vi "Roller Loop.vi"(11 "Reset Pots?":bool) -> (3 "first run complete?":bool)   [LabVIEW 2014]
uses:
  Common Code/Roller Indicators.ctl
  Common Code/Roller Mode Enum.ctl
  Common Code/Auto Roller Commands.ctl
  Common Code/Inner Roller States.ctl
  Sensors/Pot Data.ctl
  Untip Can States.ctl
  Roller Modes.ctl
  Really Real Manual Align.ctl
  Common Code/Change Detect Int.vi
  Robot Global Data.vi
  <vilib>/Rock Robotics/WPI/Solenoid/Deprecated/WPI_SolenoidSetBool.vi
  <vilib>/Rock Robotics/WPI/DriverStation/WPI_DriverStationRobotMode2.ctl
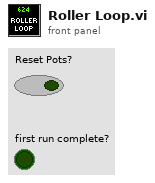
[diagram p1: front panel]
types:
  T1 = typedef "Roller Modes.ctl" = cluster{"Auto Roller Command":T2, "Roller Mode":T3, "Override Speed":dbl}
  T2 = typedef "Auto Roller Commands.ctl" = enum16{"Drag Tote", "Grab Tote", "Idle", "Eject Tote", "Untip Can", "Grab Can"}
  T3 = typedef "Roller Mode Enum.ctl" = enum16{"Manual", "Safe", "Auto"}
  T4 = typedef "Inner Roller States.ctl" = enum16{"Turn Tote Portrait", "Acquire Tote", "Absorb Tote", "Turn Tote Right", "Turn Tote Left", "Acquire Can", "Absorb Can", "Turn Can", "Hold Tote"}
  T5 = typedef "Roller Indicators.ctl" = cluster{"Rollers Closed?":bool, "Roller Mode":T3, "Auto Roller State":T2, "Tote Inside?":bool, "Intake State":T4, "Left Ping Dist":sgl, "Right Ping Dist":sgl, "Potentiometer Cluster":T6, "PING Decision":T4, "Zero Complete?":bool, "Left Arm Closed?":bool, "Portrait?":bool, "Right Arm Closed?":bool, "Left Out":sgl, "Right Out":sgl, "Left Current":sgl, "Right Current":sgl, "Tote Load Complete?":bool, "Untip Complete?":bool, "Untip State":T7, "Roller Safety Open":bool}
  T6 = typedef "Pot Data.ctl" = cluster{"Left Pot Zero":sgl, "Right Pot Zero":sgl, "Left Potentiometer":sgl, "Right Potentiometer":sgl, "Left Pot Non Zero":sgl, "Right Pot Non Zero":sgl}
  T7 = typedef "Untip Can States.ctl" = enum16{"Release Can", "Catch Can", "Idle"}
  T8 = typedef "Dashboard Control Data.ctl" = cluster{"Cam Exposure":dbl, "Go to angle":dbl, "Steer PID Gains":cluster{"proportional gain (Kc)":dbl, "integral time (Ti, min)":dbl, "derivative time (Td, min)":dbl}, "Steer PID output Range":cluster{"output high":dbl, "output low":dbl}, "Pressure m \nValue":dbl, "Pressure b \nValue":dbl, "Roller Command Cluster ":T9, "Elevator":T10, "Encoder Control":T12, "Auton Settings":cluster{"Drive Dist Window Size":dbl}, "Drivetrain Settings":T13}
  T9 = typedef "Roller Control.ctl" = cluster{"Intake Speed":dbl, "Turn In Speed":dbl, "Unload Speed":dbl, "Turn Out Speed":dbl, "Ping Align Tolerance":dbl, "Tote Range Threshold":dbl, "Right Pot 0":dbl, "Pot Threshold":dbl, "Left Pot 0":dbl, "Manual 0s?":bool, "Right Pot Scale":dbl, "Left Pot Scale":dbl, "0 wait time":i32, "Zero Pots":bool, "Min Elevator Height":dbl, "Eject Time":dbl, "Eject US Threshold":dbl, "Anti-Twitch Time":u32, "Ping Caring Threshold":dbl, "Pot Diff Threshold":dbl, "Pinch Sustain":u32, "Absorb Give Up Threshold":dbl, "Untip In Threshold":dbl, "Untip Grab Range":dbl, "Ultrasonic Hold Time":u32, "Landscape Absorb Time":u32, "Pot Use Wait Time":u32, "Can Turn Stop Range":dbl}
  T10 = typedef "Elevator DB Control.ctl" = cluster{"PID Output Range":cluster{"output high":dbl, "output low":dbl}, "PID gains":cluster{"proportional gain (Kc)":dbl, "integral time (Ti, min)":dbl, "derivative time (Td, min)":dbl}, "Height Tolerance":sgl, " Encoder Constant":dbl, "Safe Mode Max Speed":sgl, "Eject Time":sgl, "Zeroing Speed":sgl, "Presets":T11, "Ping Detect Threshold":sgl, "Trashcan Detect Threshold":sgl, "Zero Filter Time":dbl, "Stabilizer Open Time":dbl, "Zero Creep Speed":dbl, "Max Current":dbl, "Current Trip Time":dbl, "Abort Pitch":dbl}
  T11 = typedef "Elevator Presets.ctl" = cluster{"Pickup 2 w/ Tote":sgl, "Pickup 2 w/ Trashcan":sgl, "Pickup 3 w/ Tote":sgl, "Pickup 3 w/ Trashcan":sgl, "Bottom":sgl, "Pickup 1 w/ Tote":sgl, "Pickup Trashcan":sgl, "Pickup 1 w/ Trashcan":sgl, "Eject":sgl, "Hold Low":sgl, "Step add height":sgl, "Store Trashcan 3":sgl, "Store Trashcan 4":sgl, "Store Trashcan 5":sgl, "6 Tote Max":sgl, "5 Tote Max":sgl, "Untip Lift":dbl, "Drop Stack":dbl, "Pickup 1 Empty":dbl, "Pickup 2 Empty":dbl, "Pickup 3 Empty":dbl, "4 Tote Max":dbl, "HP Load Hold":dbl, "HP Load Drop":dbl, "HP Load Finger":dbl}
  T12 = typedef "Encoder Control.ctl" = cluster{"Left Tick Constant":dbl, "Right Tick Constant":dbl, "Center Tick Constant":dbl, "Reset?":bool, "Y Dist":cluster{"PID gains":cluster{"proportional gain (Kc)":dbl, "integral time (Ti, min)":dbl, "derivative time (Td, min)":dbl}}, "X Dist":cluster{"PID gains":cluster{"proportional gain (Kc)":dbl, "integral time (Ti, min)":dbl, "derivative time (Td, min)":dbl}}, "Y Stop Thresh":dbl, "Y Stop Speed":dbl, "X Stop Thresh":dbl, "X Stop Speed":dbl}
  T13 = typedef "Drivetrain Settings.ctl" = cluster{"Gyro Tolerance":dbl, "Strafe Correct max steer":dbl, "Strafe Timer Wait":dbl, "Throttle Ramp (ms)":dbl, "Strafe Ramp (ms)":dbl}
  T14 = typedef "Ultrasonic Indicators.ctl" = cluster{"Left Distance":dbl, "Right Distance":dbl, "Center Distance":dbl, "Left Distance Unfilter":dbl, "Right Distance Unfilter":dbl, "Center Distance Unfilter":dbl}
  T15 = typedef "Roller Manual Bools.ctl" = cluster{"Manual Claw":bool, "Left Roller":bool, "Right Roller":bool, "Left Roller Back":bool, "Right Roller Back":bool, "Manual Align":T16}
  T16 = typedef "Really Real Manual Align.ctl" = enum16{"In", "Left", "Right", "Out", "Idle"}
  T17 = typedef "Elevator Status.ctl" = cluster{"Eject Piston":bool, "Height":dbl, "Top Limit":bool, "Bottom Limit":bool, "Enc Value":dbl, "Limit Override":bool, "Mode":T18, "Stabilizer":bool, "Finger":bool, "High IR":bool, "Motor Out":dbl, "Ping Detect":bool, "Auto Elevator Indicators":T19, "Master Current":dbl, "Slave Current":dbl, "High Current":bool, "Current Tripped":bool}
  T18 = typedef "Elevator Mode.ctl" = enum16{"Manual", "Safe", "Auto"}
  T19 = typedef "Auto Elevator Indicators.ctl" = cluster{"Target Out":dbl, "Storing Trashcan?":bool, "State":T20, "In Range":bool, "Store Can Command":bool, "HP Load":bool}
  T20 = typedef "Elevator State.ctl" = enum16{"Idle", "Goto Load Position", "Wait for Load", "Load Drop", "Load Lift", "Drop Stack", "Goto Eject Position", "Eject ", "Raise Trashcan", "Open Stabilizer", "Untip Drop", "Untip Wait", "Untip Lift", "Abort Load", "HP Load Wait", "HP Load Drop", "HP Load Lift", "HP Load Abort"}
  T21 = typedef "WPI_DriverStationRobotMode2.ctl" = enum16{"Autonomous Disabled", "Autonomous Enabled", "Teleop Disabled", "Teleop Enabled", "Disconnected", "Finish", "Test Disabled", "Test Enabled", "Emergency Stopped"}
  T22 = typedef "WPI_SolenoidDevRef.ctl" = cluster{"DevStatus":errorcluster, "Pneumatics Control Module":u8, "Forward Solenoid Channel":T23, "Reverse Solenoid Channel":T23}
  T23 = typedef "WPI_SolenoidChannel.ctl" = enum8{"Solenoid 0", "Solenoid 1", "Solenoid 2", "Solenoid 3", "Solenoid 4", "Solenoid 5", "Solenoid 6", "Solenoid 7", "Invalid"}
  T24 = typedef "WPI_MotorControlDeviceRef.ctl" = cluster{"DeviceStatus":errorcluster, "Type":T25, "PWM":cluster{"Controller":T26, "PWM Channel":T27, "DeadBand":T28}, "CAN":cluster{"Device Number":u8, "Control Mode":T29, "Semaphore":T30, "Max Vout":dbl, "TalonSRX Control Mode":T31}, "Invert":bool, "TransformRef":T32, "InvTransformRef":T32}
  T25 = typedef "WPI_MotorControlType.ctl" = enum16{"PWM", "CAN", "CANTalonSRX"}
  T26 = typedef "FPGA_TypedefDigitalModule.ctl" = enum16{"Controller 1"}
  T27 = typedef "FPGA_DIOPWMChannel.ctl" = enum8{"PWM 0", "PWM 1", "PWM 2", "PWM 3", "PWM 4", "PWM 5", "PWM 6", "PWM 7", "PWM 8", "PWM 9", "PWM MXP 0", "PWM MXP 1", "PWM MXP 2", "PWM MXP 3", "PWM MXP 4", "PWM MXP 5", "PWM MXP 6", "PWM MXP 7", "PWM MXP 8", "PWM MXP 9", "Invalid"}
  T28 = typedef "WPI_PWMDeadband.ctl" = cluster{"Name":string, "maxPositivePwm":i32, "minPositivePwm":i32, "centerPwm":i32, "maxNegativePwm":i32, "minNegativePwm":i32, "angularRange":u16}
  T29 = typedef "WPI_CANJaguar_ControlMode.ctl" = enum8{"Percent VBus", "Current", "Speed", "Position", "Voltage"}
  T30 = typedef "Semaphore RefNum" = refnum<k1>
  T31 = typedef "WPI_CANTalonSRX_APIControlMode.ctl" = enum8{"Percent VBus", "Speed", "Position", "Slave", "Unchanged / Invalid"}
  T32 = typedef "WPI_PWMTransform_ConPane.ctl" = refnum<vi>
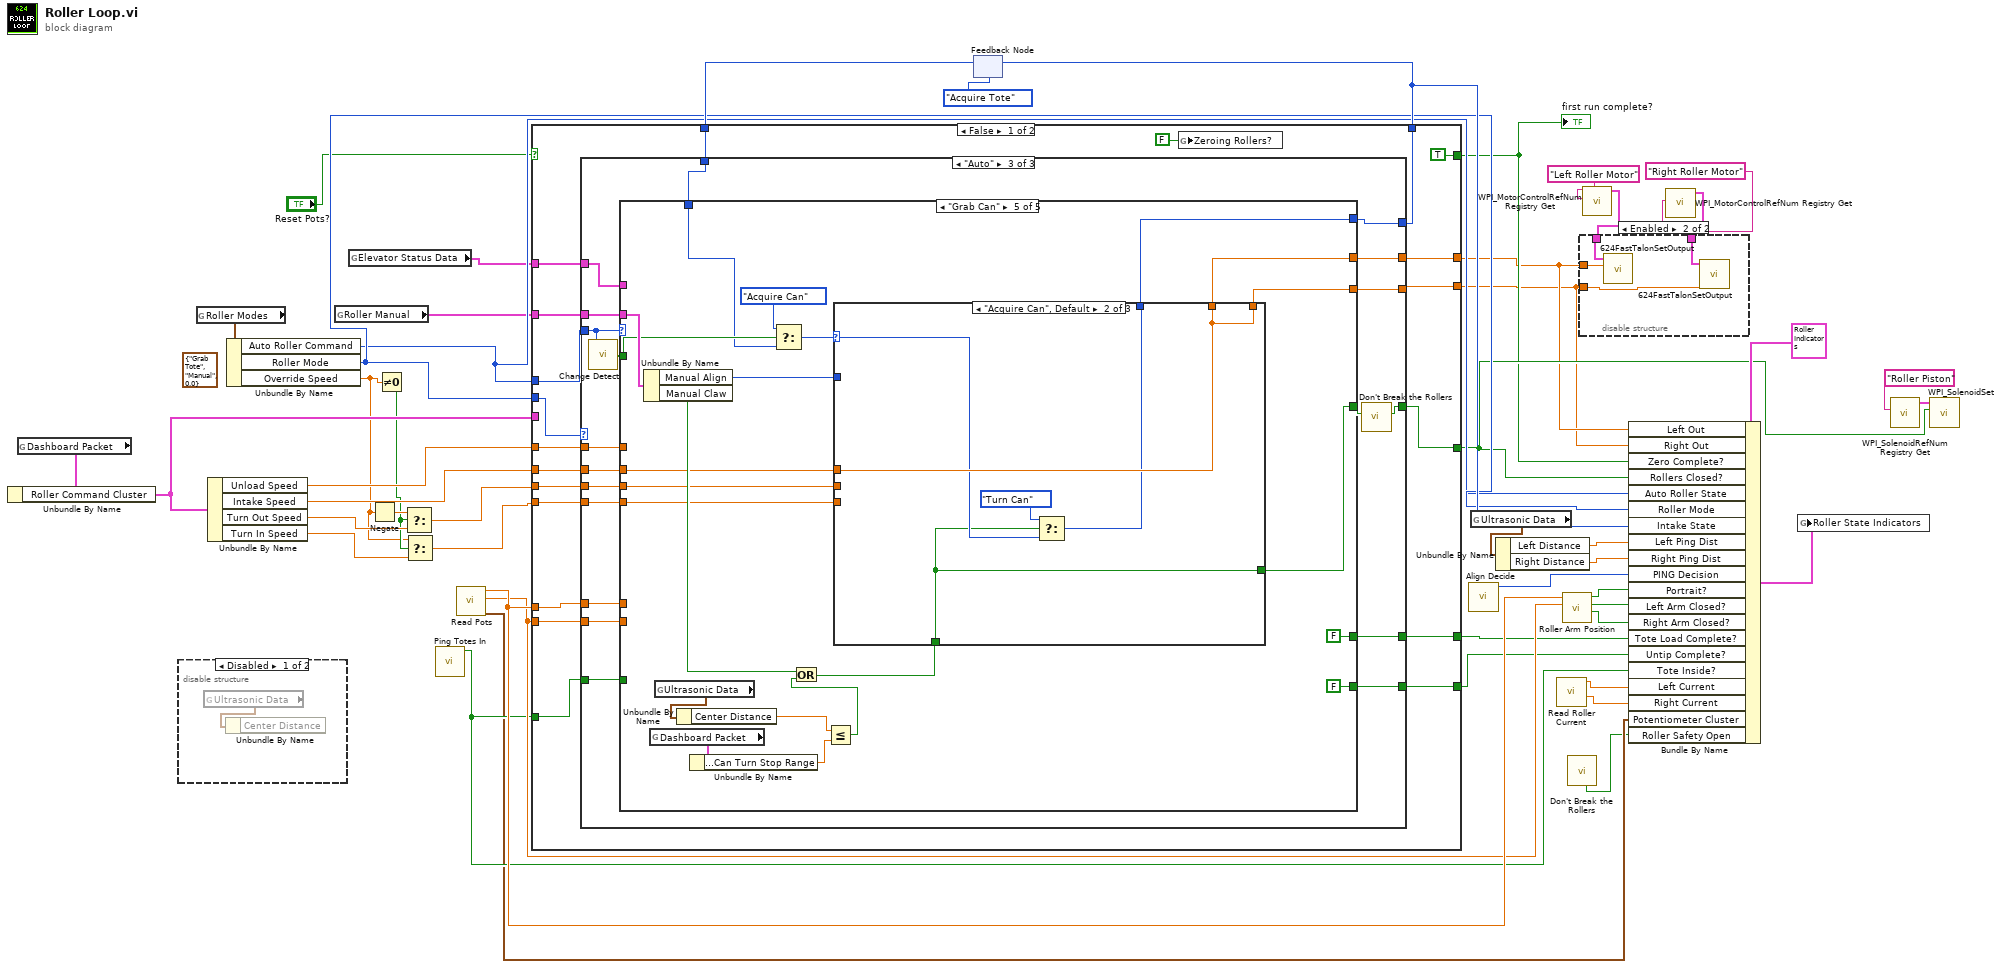
[diagram p0: block diagram]
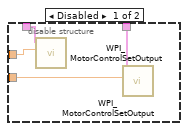
[diagram p2: hidden frame]
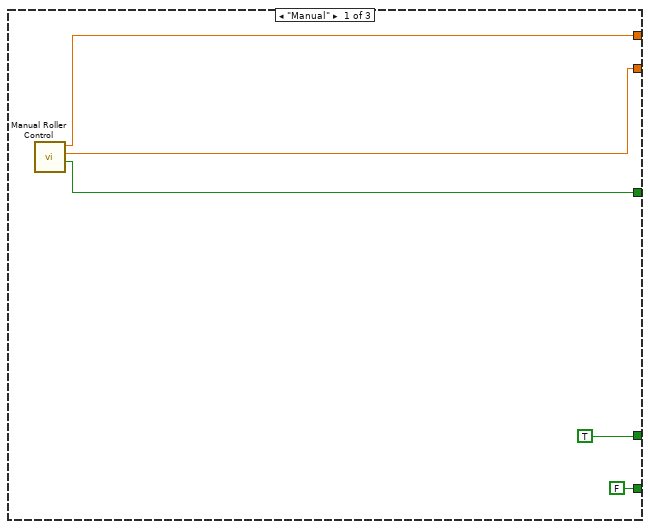
[diagram p3: hidden frame]
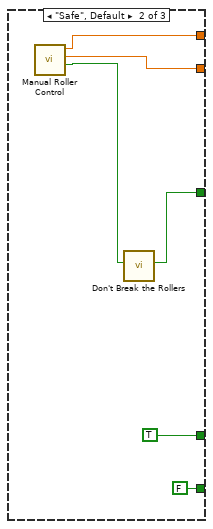
[diagram p4: hidden frame]
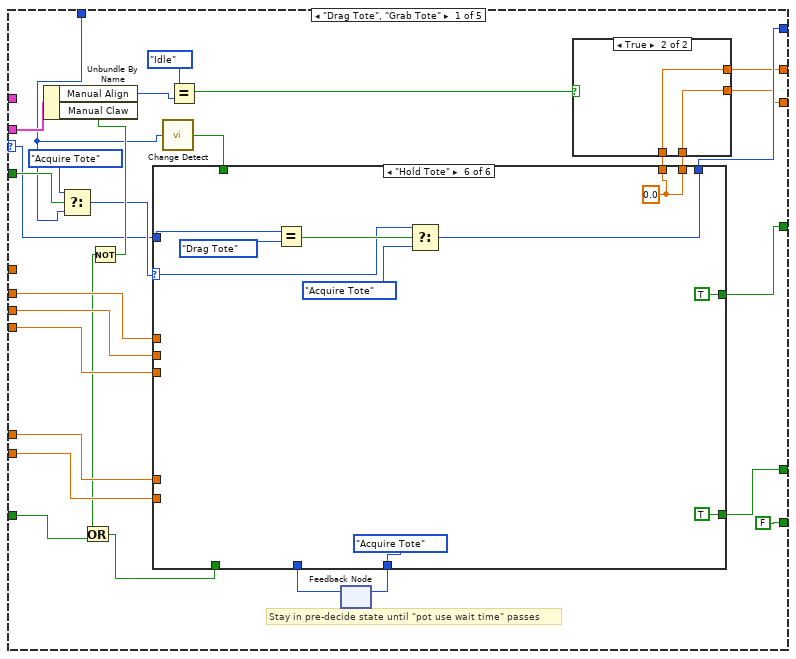
[diagram p5: hidden frame]
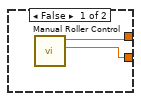
[diagram p6: hidden frame]
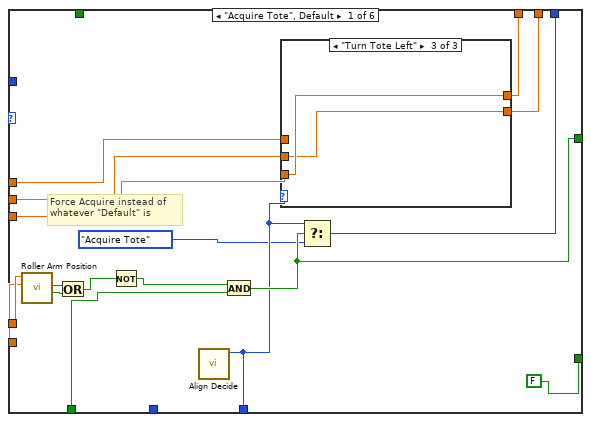
[diagram p7: hidden frame]
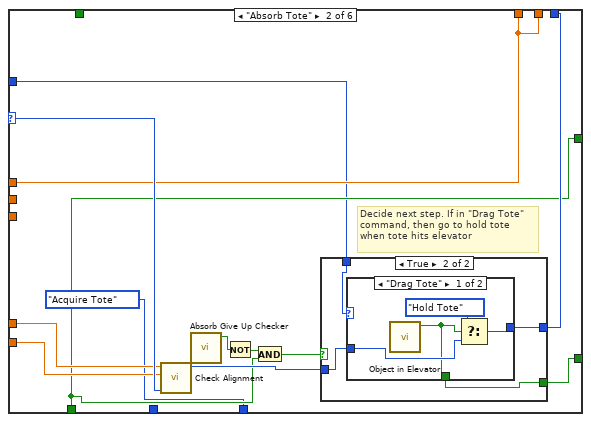
[diagram p10: hidden frame]
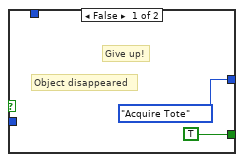
[diagram p11: hidden frame]
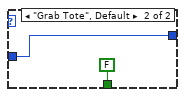
[diagram p12: hidden frame]
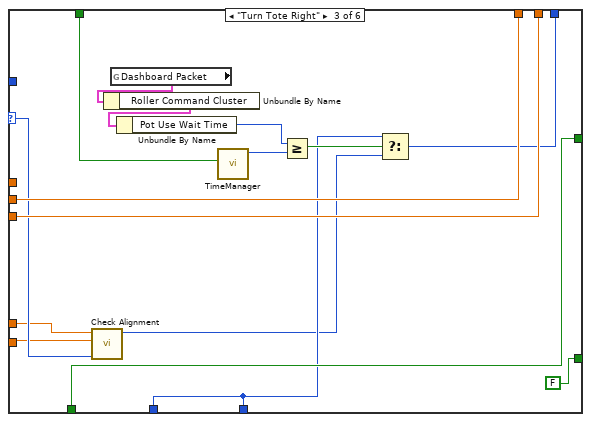
[diagram p13: hidden frame]
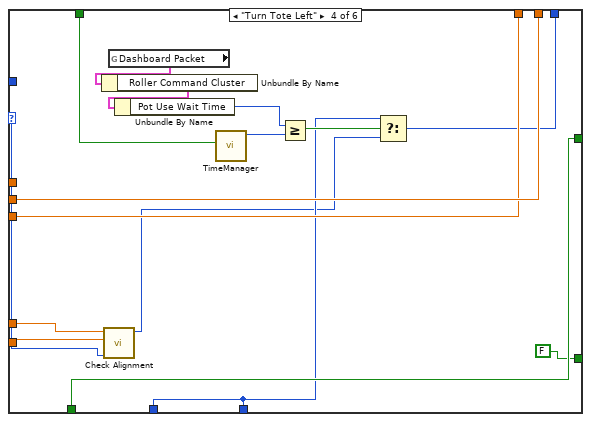
[diagram p14: hidden frame]
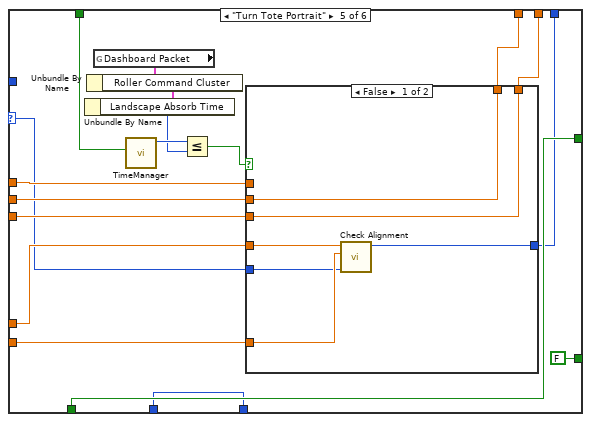
[diagram p15: hidden frame]
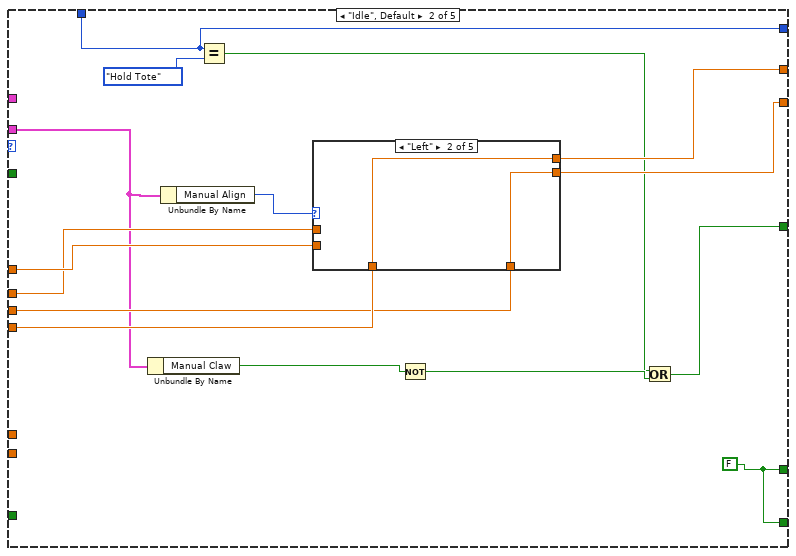
[diagram p17: hidden frame]
diagram:
  (unwired) T1 {"Auto Roller Command"=enum."Grab Tote", "Roller Mode"=enum."Manual", "Override Speed"=0.0} ("input cluster")
  n1 = global read "Robot Global Data.vi" "Dashboard Packet"() -> (w28:T8)
  n2 = Unbundle By Name(w28) -> ("Roller Command Cluster"=w29:T9)
  n3 = disable-structure shown="Disabled" {
    frame Disabled {
      n4 = global read "Robot Global Data.vi" "Ultrasonic Data"() -> (w49:T14)
      n5 = Unbundle By Name(w49) -> ()  [unwired: 1 out]
    }
    frame Enabled {
    }
  }
  n6 = global read "Robot Global Data.vi" "Roller Modes"() -> (w43:T1)
  n7 = Unbundle By Name(w29) -> ("Unload Speed"=w15:dbl, "Intake Speed"=w14:dbl, "Turn Out Speed"=w6:dbl, "Turn In Speed"=w5:dbl)
  n8 = Unbundle By Name(w43) -> ("Auto Roller Command"=w40:T2, "Roller Mode"=w41:T3, "Override Speed"=w2:dbl)
  n9 = global read "Robot Global Data.vi" "Roller Manual"() -> (w23:T15)
  n10 = global read "Robot Global Data.vi" "Elevator Status Data"() -> (w24:T17)
  n11 = Negate(x=w2) -> (-x=w7:dbl)
  n12 = Not Equal To 0?(x=w2) -> (x != 0?=w3:bool)
  n13 = Select(t=w7, s=w3, f=w6) -> (s? t:f=w8:dbl)
  n14 = Select(t=w2, s=w3, f=w5) -> (s? t:f=w4:dbl)
  n15 = call "Ping Totes In.vi"() -> ("In?"=w13:bool)  [unwired: 11 in]
  n16 = call "Read Pots.vi"() -> ("Pot Write Cluster"=w10:T6, "Right Pot"=w32:dbl, "Left Pot"=w33:dbl)  [unwired: 7 in, 2 out]
  n17 = feedback #1(Inner_Roller_States."Acquire Tote" ("Enum")) -> (w47:T4)
  n18 = case shown="False" "Reset Pots?" {
    tunnel: w14 -> [w69 _]
    tunnel: w8 -> [w68 _]
    tunnel: w4 -> [w67 _]
    tunnel: w47 -> [w66 w376]
    tunnel: [w65 FALSE ("Manual Claw")] -> w38
    tunnel: w23 -> [w64 _]
    tunnel: [w63 0.0 ("Left Roller Speed Unload")] -> w31
    tunnel: [w62 0.0 ("Right Roller Speed Unload")] -> w30
    tunnel: w15 -> [w61 _]
    tunnel: [w60 w376] -> w42
    tunnel: w41 -> [w59 _]
    tunnel: w40 -> [w58 _]
    tunnel: w13 -> [w57 _]
    tunnel: w29 -> [_ w377]
    tunnel: [TRUE w375] -> w37
    tunnel: w33 -> [w55 _]
    tunnel: w32 -> [w54 _]
    tunnel: [w53 w373] -> w27
    tunnel: w24 -> [w52 _]
    tunnel: [w51 w373] -> w26
    frame False {
      n19 = case shown="\"Auto\"" w59 {
        tunnel: w64 -> [_ _ w90]
        tunnel: w69 -> [_ _ w98]
        tunnel: w68 -> [_ _ w96]
        tunnel: w67 -> [_ _ w97]
        tunnel: w58 -> [_ _ w81]
        tunnel: [_ _ w94] -> w60
        tunnel: w66 -> [_ _ w99]
        tunnel: [w70 w80 w87] -> w65
        tunnel: w57 -> [_ _ w95]
        tunnel: [w72 w77 w93] -> w63
        tunnel: [w71 w76 w92] -> w62
        tunnel: w61 -> [_ _ w91]
        tunnel: w55 -> [_ _ w89]
        tunnel: w54 -> [_ _ w88]
        tunnel: [TRUE TRUE w85] -> w53
        tunnel: w52 -> [_ _ w84]
        tunnel: [FALSE FALSE w82] -> w51
        frame "Manual" {
          n20 = call "Manual Roller Control.vi"() -> ("Boolean"=w70:bool, "Right Speed Out"=w71:dbl, "Left Speed Out"=w72:dbl)  [unwired: 9 in]
        }
        frame "Safe", Default {
          n21 = call "Manual Roller Control.vi"() -> ("Boolean"=w75:bool, "Right Speed Out"=w76:dbl, "Left Speed Out"=w77:dbl)  [unwired: 9 in]
          n22 = call "Don't Break the Rollers.vi"("Rollers close in"=w75) -> ("Roller close out"=w80:bool)  [unwired: 9 in, 1 out]
        }
        frame "Auto" {
          n23 = call-poly "Change Detect.vi"("In"=w81) -> ("Changed?"=w83:bool)
          n24 = case shown="\"Grab Can\"" w81 {
            selector: w81 -> [w100 _ w273 _ _]
            tunnel: w99 -> [w103 w248 w275 w286 w336]
            tunnel: [w128 w249 w270 w278 w323] -> w86
            tunnel: w98 -> [w127 w261 _ w284 w332]
            tunnel: w97 -> [w126 w257 _ _ w330]
            tunnel: w96 -> [w125 w256 _ _ w331]
            tunnel: w95 -> [w118 _ _ _ _]
            tunnel: [w112 w248 w275 w286 w327] -> w94
            tunnel: [w111 w260 w272 w279 w328] -> w93
            tunnel: [w108 w259 w271 w279 w329] -> w92
            tunnel: w91 -> [_ w262 _ _ _]
            tunnel: w90 -> [w121 w255 _ _ w339]
            tunnel: w89 -> [w124 _ _ _ _]
            tunnel: w88 -> [w123 _ _ _ _]
            tunnel: [w122 w253 w274 FALSE FALSE] -> w85
            tunnel: w84 -> [_ _ _ w287 _]
            tunnel: w83 -> [w104 _ _ w283 w337]
            tunnel: [FALSE w253 w274 w277 FALSE] -> w82
            frame "Drag Tote", "Grab Tote" {
              # "Stay in pre-decide state until \"pot use wait time\" passes"
              n25 = Unbundle By Name(w121) -> ("Manual Align"=w115:T16, "Manual Claw"=w120:bool)
              n26 = Select(t=Inner_Roller_States."Acquire Tote", s=w104, f=w103) -> (s? t:f=w101:T4)
              n27 = Not(x=w120) -> (.not. x?=w119:bool)
              n28 = Or(x=w119, y=w118) -> (x .or. y?=w117:bool)
              n29 = call-poly "Change Detect.vi"("In"=w103) -> ("Changed?"=w107:bool)
              n30 = Equal?(x=Really_Real_Manual_Align."Idle" ("y"), y=w115) -> (x = y?=w113:bool)
              n31 = feedback #2() -> (w105:T4)  [unwired: 1 in]
              n32 = case shown="\"Hold Tote\"" w101 {
                selector: w101 -> [_ w165 w193 w211 w217 w240]
                tunnel: w117 -> [w139 w159 w190 w206 w223 _]
                tunnel: [w138 w159 w190 w206 w223 TRUE] -> w128
                tunnel: [w149 w167 w180 w198 w216 w238] -> w112
                tunnel: w127 -> [w148 w162 _ _ w226 _]
                tunnel: w126 -> [w147 _ w195 w207 w220 _]
                tunnel: w125 -> [w146 _ w194 w208 w221 _]
                tunnel: [w145 w162 w194 w207 w225 w247] -> w110
                tunnel: [w144 w162 w195 w208 w224 w247] -> w109
                tunnel: w124 -> [w143 w164 w192 w210 w218 _]
                tunnel: w123 -> [w142 w163 w191 w209 w219 _]
                tunnel: [FALSE w161 FALSE FALSE FALSE TRUE ("Boolean")] -> w122
                tunnel: w107 -> [_ _ w186 w201 w229 _]
                tunnel: [w134 Inner_Roller_States."Acquire Tote" ("Next Step") w182 w200 w212 Inner_Roller_States."Acquire Tote" ("Next Step")] -> w106
                tunnel: w105 -> [_ _ w182 w200 w212 _]
                tunnel: w100 -> [_ w155 _ _ _ w243]
                frame "Acquire Tote", Default {
                  # "Force Acquire instead of \nwhatever \"Default\" is"
                  n33 = call "Roller Arm Position.vi"("Right Pot"=w142, "Left Pot"=w143) -> ("Right Closed?"=w141:bool, "Left Closed?"=w140:bool)  [unwired: 6 in, 2 out]
                  n34 = Or(x=w140, y=w141) -> (x .or. y?=w137:bool)
                  n35 = Not(x=w137) -> (.not. x?=w136:bool)
                  n36 = call "Align Decide.vi"() -> ("Next Step"=w134:T4)  [unwired: 11 in]
                  n37 = And(x=w136, y=w139) -> (x .and. y?=w138:bool)
                  n38 = case shown="\"Turn Tote Left\"" w134 {
                    tunnel: w148 -> [w150 _ _]
                    tunnel: w147 -> [_ w152 w154]
                    tunnel: w146 -> [_ w151 w153]
                    tunnel: [w150 w151 w154] -> w145
                    tunnel: [w150 w152 w153] -> w144
                    frame "Absorb Tote", Default {
                    }
                    frame "Turn Tote Right" {
                    }
                    frame "Turn Tote Left" {
                    }
                  }
                  n39 = Select(t=w134, s=w138, f=Inner_Roller_States."Acquire Tote") -> (s? t:f=w149:T4)
                }
                frame "Absorb Tote" {
                  # "Decide next step. If in \"Drag Tote\"\ncommand, then go to hold tote\nwhen tote hits elevator"
                  n40 = call "Check Alignment.vi"("Current State"=w165, "Right Pot"=w163, "Left Pot"=w164) -> ("State Output"=w166:T4)  [unwired: 8 in]
                  n41 = call "Absorb Give Up Checker.vi"() -> ("Give Up?"=w160:bool)  [unwired: 11 in]
                  n42 = Not(x=w160) -> (.not. x?=w158:bool)
                  n43 = And(x=w158, y=w159) -> (x .and. y?=w157:bool)
                  n44 = case shown="True" w157 {
                    tunnel: [Inner_Roller_States."Acquire Tote" ("State Output") w171] -> w167
                    tunnel: w166 -> [_ w172]
                    tunnel: [TRUE w170] -> w161
                    tunnel: w155 -> [_ w173]
                    frame False {
                      # "Object disappeared"
                      # "Give up!"
                    }
                    frame True {
                      n45 = case shown="\"Drag Tote\"" w173 {
                        tunnel: w172 -> [w177 w179]
                        tunnel: [w176 w179] -> w171
                        tunnel: [w174 FALSE ("Boolean")] -> w170
                        frame "Drag Tote" {
                          n46 = call "Object in Elevator.vi"() -> ("Boolean"=w174:bool)  [unwired: 11 in]
                          n47 = Select(t=Inner_Roller_States."Hold Tote", s=w174, f=w177) -> (s? t:f=w176:T4)
                        }
                        frame "Grab Tote", Default {
                        }
                      }
                    }
                  }
                }
                frame "Turn Tote Right" {
                  n48 = call "Check Alignment.vi"("Current State"=w193, "Right Pot"=w191, "Left Pot"=w192) -> ("State Output"=w181:T4)  [unwired: 8 in]
                  n49 = global read "Robot Global Data.vi" "Dashboard Packet"() -> (w188:T8)
                  n50 = Unbundle By Name(w188) -> ("Roller Command Cluster"=w187:T9)
                  n51 = Unbundle By Name(w187) -> ("Pot Use Wait Time"=w184:u32)
                  n52 = call "TimeManager.vi"("Reset?"=w186) -> ("Time Since Reset"=w185:u32)  [unwired: 9 in, 1 out]
                  n53 = Greater Or Equal?(x=w184, y=w185) -> (x >= y?=w183:bool)
                  n54 = Select(t=w182, s=w183, f=w181) -> (s? t:f=w180:T4)
                }
                frame "Turn Tote Left" {
                  n55 = call "Check Alignment.vi"("Current State"=w211, "Right Pot"=w209, "Left Pot"=w210) -> ("State Output"=w199:T4)  [unwired: 8 in]
                  n56 = global read "Robot Global Data.vi" "Dashboard Packet"() -> (w196:T8)
                  n57 = Unbundle By Name(w196) -> ("Roller Command Cluster"=w197:T9)
                  n58 = Unbundle By Name(w197) -> ("Pot Use Wait Time"=w203:u32)
                  n59 = call "TimeManager.vi"("Reset?"=w201) -> ("Time Since Reset"=w202:u32)  [unwired: 9 in, 1 out]
                  n60 = Greater Or Equal?(x=w203, y=w202) -> (x >= y?=w204:bool)
                  n61 = Select(t=w200, s=w204, f=w199) -> (s? t:f=w198:T4)
                }
                frame "Turn Tote Portrait" {
                  n62 = global read "Robot Global Data.vi" "Dashboard Packet"() -> (w215:T8)
                  n63 = Unbundle By Name(w215) -> ("Roller Command Cluster"=w214:T9)
                  n64 = Unbundle By Name(w214) -> ("Landscape Absorb Time"=w213:u32)
                  n65 = call "TimeManager.vi"("Reset?"=w229) -> ("Time Since Reset"=w228:u32)  [unwired: 9 in, 1 out]
                  n66 = Less Or Equal?(x=w228, y=w213) -> (x <= y?=w227:bool)
                  n67 = case shown="False" w227 {
                    tunnel: [w235 w237] -> w225
                    tunnel: w226 -> [_ w237]
                    tunnel: [w234 w237] -> w224
                    tunnel: w221 -> [w235 _]
                    tunnel: w220 -> [w234 _]
                    tunnel: w219 -> [w233 _]
                    tunnel: w218 -> [w232 _]
                    tunnel: w217 -> [w231 w236]
                    tunnel: [w230 w236] -> w216
                    frame False {
                      n68 = call "Check Alignment.vi"("Current State"=w231, "Right Pot"=w233, "Left Pot"=w232) -> ("State Output"=w230:T4)  [unwired: 8 in]
                    }
                    frame True {
                    }
                  }
                }
                frame "Hold Tote" {
                  w247 = 0.0
                  n69 = Equal?(x=w243, y=Auto_Roller_Commands."Drag Tote") -> (x = y?=w241:bool)
                  n70 = Select(t=w240, s=w241, f=Inner_Roller_States."Acquire Tote") -> (s? t:f=w238:T4)
                }
              }
              n71 = feedback-in #2(w106) -> ()
              n72 = case shown="True" w113 {
                tunnel: [w130 w132] -> w111
                tunnel: w110 -> [_ w132]
                tunnel: [w129 w131] -> w108
                tunnel: w109 -> [_ w131]
                frame False {
                  n73 = call "Manual Roller Control.vi"() -> ("Right Speed Out"=w129:dbl, "Left Speed Out"=w130:dbl)  [unwired: 9 in, 1 out]
                }
                frame True {
                }
              }
            }
            frame "Idle", Default {
              w253 = FALSE
              n74 = Unbundle By Name(w255) -> ("Manual Claw"=w254:bool)
              n75 = Unbundle By Name(w255) -> ("Manual Align"=w258:T16)
              n76 = Equal?(x=w248, y=Inner_Roller_States."Hold Tote") -> (x = y?=w250:bool)
              n77 = case shown="\"Left\"" w258 {
                tunnel: [w263 w265 w267 w268 w269] -> w259
                tunnel: w261 -> [w263 _ _ _ _]
                tunnel: [w263 w264 w266 w268 w269] -> w260
                tunnel: w262 -> [_ _ _ w268 _]
                tunnel: w256 -> [_ w265 w266 _ _]
                tunnel: w257 -> [_ w264 w267 _ _]
                frame "In", Default {
                }
                frame "Left" {
                }
                frame "Right" {
                }
                frame "Out" {
                }
                frame "Idle" {
                  w269 = 0.0 ("Unload Speed")
                }
              }
              n78 = Not(x=w254) -> (.not. x?=w251:bool)
              n79 = Or(x=w250, y=w251) -> (x .or. y?=w249:bool)
            }
            frame "Eject Tote" {
              w274 = FALSE
              n80 = call-poly "Change Detect.vi"("In"=w273) -> ()  [unwired: 1 out]
              n81 = call "Roller Step Eject.vi"() -> ("Close Rollers?"=w270:bool, "Right Out"=w271:dbl, "Left Out"=w272:dbl)  [unwired: 9 in]
            }
            frame "Untip Can" {
              n82 = feedback #3(Untip_Can_States."Idle") -> (w282:T7)
              n83 = Select(t=Untip_Can_States."Idle", s=w283, f=w282) -> (s? t:f=w281:T7)
              n84 = case shown="\"Release Can\"" w281 {
                selector: w281 -> [w289 w300 w314]
                tunnel: w287 -> [_ _ w310]
                tunnel: w284 -> [_ w303 w317]
                tunnel: [0.0 ("Intake Speed") w303 w317] -> w279
                tunnel: [FALSE TRUE FALSE] -> w278
                tunnel: [TRUE FALSE FALSE] -> w277
                tunnel: [w289 w299 w313] -> w276
                frame "Release Can" {
                }
                frame "Catch Can" {
                  n85 = global read "Robot Global Data.vi" "Dashboard Packet"() -> (w296:T8)
                  n86 = global read "Robot Global Data.vi" "Ultrasonic Data"() -> (w294:T14)
                  n87 = Unbundle By Name(w294) -> ("Center Distance"=w295:dbl)
                  n88 = Unbundle By Name(w296) -> ("Roller Command Cluster.Untip In Threshold"=w297:dbl)
                  n89 = Less Or Equal?(x=w295, y=w297) -> (x <= y?=w298:bool)
                  n90 = Select(t=Untip_Can_States."Release Can", s=w298, f=w300) -> (s? t:f=w299:T7)
                }
                frame "Idle", Default {
                  n91 = global read "Robot Global Data.vi" "Dashboard Packet"() -> (w305:T8)
                  n92 = global read "Robot Global Data.vi" "Ultrasonic Data"() -> (w307:T14)
                  n93 = Unbundle By Name(w305) -> ("Roller Command Cluster.Untip Grab Range"=w306:dbl)
                  n94 = Unbundle By Name(w307) -> ("Center Distance"=w308:dbl)
                  n95 = Unbundle By Name(w310) -> ("Auto Elevator Indicators.In Range"=w311:bool)
                  n96 = Less Or Equal?(x=w308, y=w306) -> (x <= y?=w309:bool)
                  n97 = And(x=w311, y=w309) -> (x .and. y?=w312:bool)
                  n98 = Select(t=Untip_Can_States."Catch Can", s=w312, f=w314) -> (s? t:f=w313:T7)
                }
              }
              n99 = feedback-in #3(w276) -> ()
            }
            frame "Grab Can" {
              n100 = Unbundle By Name(w339) -> ("Manual Align"=w333:T16, "Manual Claw"=w338:bool)
              n101 = global read "Robot Global Data.vi" "Dashboard Packet"() -> (w321:T8)
              n102 = global read "Robot Global Data.vi" "Ultrasonic Data"() -> (w322:T14)
              n103 = Unbundle By Name(w322) -> ("Center Distance"=w320:dbl)
              n104 = Unbundle By Name(w321) -> ("Roller Command Cluster.Can Turn Stop Range"=w319:dbl)
              n105 = Select(t=Inner_Roller_States."Acquire Can", s=w337, f=w336) -> (s? t:f=w334:T4)
              n106 = Less Or Equal?(x=w320, y=w319) -> (x <= y?=w318:bool)
              n107 = Or(x=w338, y=w318) -> (x .or. y?=w326:bool)
              n108 = case shown="\"Acquire Can\", Default" w334 {
                selector: w334 -> [w342 w348 w357]
                tunnel: w333 -> [_ _ w358]
                tunnel: [w344 w349 w353] -> w328
                tunnel: w332 -> [w344 w349 w351]
                tunnel: w331 -> [_ _ w354]
                tunnel: w330 -> [_ _ w352]
                tunnel: [w344 w349 w355] -> w329
                tunnel: [w341 w346 w356] -> w327
                tunnel: w326 -> [w343 w345 _]
                tunnel: [w343 w345 TRUE] -> w323
                frame "Absorb Can" {
                  n109 = Select(t=w342, s=w343, f=Inner_Roller_States."Acquire Can") -> (s? t:f=w341:T4)
                }
                frame "Acquire Can", Default {
                  n110 = Select(t=Inner_Roller_States."Turn Can", s=w345, f=w348) -> (s? t:f=w346:T4)
                }
                frame "Turn Can" {
                  n111 = case shown="\"In\", Default" w358 {
                    tunnel: w357 -> [_ w363 w366]
                    tunnel: [Inner_Roller_States."Absorb Can" ("t") w363 w366] -> w356
                    tunnel: [w359 w362 w364] -> w355
                    tunnel: w354 -> [_ w362 w365]
                    tunnel: [w359 w361 w365] -> w353
                    tunnel: w352 -> [_ w361 w364]
                    tunnel: w351 -> [w359 _ _]
                    frame "In", Default {
                    }
                    frame "Left" {
                    }
                    frame "Right" {
                    }
                  }
                }
              }
            }
          }
          n112 = call "Don't Break the Rollers.vi"("Rollers close in"=w86) -> ("Roller close out"=w87:bool)  [unwired: 9 in, 1 out]
        }
      }
      n113 = global write "Robot Global Data.vi" "Zeroing Rollers?"(FALSE ("Zeroing Rollers?")) -> ()
    }
    frame True {
      w373 = FALSE
      n114 = disable-structure shown="Enabled" {
        disable-tunnel: [w385 TRUE] -> w371
        frame Disabled {
          n115 = call <vilib>:"WPI_DriverStationGetModeAndStatus.vi"() -> ("Robot Mode"=w383:T21)  [unwired: 10 in, 1 out]
          n116 = Equal?(x=w383, y=WPI_DriverStationRobotMode2."Teleop Enabled") -> (x = y?=w382:bool)
          n117 = Equal?(x=WPI_DriverStationRobotMode2."Autonomous Enabled", y=w383) -> (x = y?=w384:bool)
          n118 = Or(x=w384, y=w382) -> (x .or. y?=w385:bool)
        }
        frame Enabled {
        }
      }
      n119 = disable-structure shown="Disabled" {
        frame Disabled {
          # "wait until it's safe to close rollers"
          n120 = call "Don't Break the Rollers.vi"() -> ()  [unwired: 10 in, 2 out]
          n121 = call "Don't Break the Rollers.vi"() -> ("Keeep rollers open?"=w401:bool)  [unwired: 10 in, 1 out]
          n122 = Not(x=w401) -> ()  [unwired: 1 out]
        }
        frame Enabled {
        }
      }
      n123 = call "Get Pressure.vi"() -> ("Pressure"=w369:dbl)  [unwired: 10 in, 1 out]
      n124 = Greater Or Equal?(x=w369, y=60.0) -> (x >= y?=w370:bool)
      n125 = Compound Arithmetic op=AND(w370, w371) -> (w372:bool)
      n126 = case shown="True" w372 {
        tunnel: w377 -> [_ w390]
        tunnel: [FALSE w388] -> w375
        frame False {
        }
        frame True {
          n127 = flat-sequence {
            tunnel: w389 -> [w392]
            tunnel: [TRUE] -> w388
            frame #0 {
              # "Close"
              n128 = call <vilib>:"WPI_SolenoidRefNum Registry Get.vi"("refnum name"="Roller Piston") -> ("SolenoidDevRef"=w394:T22)  [unwired: 9 in, 1 out]
              n129 = call-poly <vilib>:"WPI_SolenoidSet.vi"("Value"=FALSE, "SolenoidDevRef"=w394) -> ()  [unwired: 8 in, 2 out]
              n130 = Wait (ms)(milliseconds to wait=w392) -> ()  [unwired: 1 out]
            }
            frame #1 {
              w395 = 20.0 ("y")
              n131 = call "Read Pots.vi"() -> ("Unzeroed Right Pot"=w399:dbl, "Unzeroed Left Pot"=w397:dbl)  [unwired: 7 in, 3 out]
              n132 = Subtract(x=w399, y=w395) -> (x-y=w398:dbl)
              n133 = Subtract(x=w397, y=w395) -> (x-y=w396:dbl)
              n134 = global write "Robot Global Data.vi" "Left Pot 0"(w396) -> ()
              n135 = global write "Robot Global Data.vi" "Right Pot 0"(w398) -> ()
            }
          }
          n136 = Unbundle By Name(w390) -> ("0 wait time"=w389:i32)
        }
      }
      n137 = global write "Robot Global Data.vi" "Zeroing Rollers?"(TRUE ("Zeroing Rollers?")) -> ()
    }
  }
  "first run complete?" <- w37
  n138 = feedback-in #1(w42) -> ()
  n139 = call "Align Decide.vi"() -> ("Next Step"=w39:T4)  [unwired: 11 in]
  n140 = global read "Robot Global Data.vi" "Ultrasonic Data"() -> (w16:T14)
  n141 = Unbundle By Name(w16) -> ("Left Distance"=w18:dbl, "Right Distance"=w17:dbl)
  n142 = call "Read Roller Current.vi"() -> ("R Current"=w11:dbl, "L Current"=w12:dbl)  [unwired: 10 in]
  n143 = call "Roller Arm Position.vi"("Right Pot"=w32, "Left Pot"=w33) -> ("Right Closed?"=w34:bool, "Left Closed?"=w35:bool, "Portrait?"=w36:bool)  [unwired: 6 in, 1 out]
  n144 = call "Don't Break the Rollers.vi"() -> ("Keeep rollers open?"=w1:bool)  [unwired: 10 in, 1 out]
  n145 = call <vilib>:"WPI_MotorControlRefNum Registry Get.vi"("refnum name"="Left Roller Motor") -> ("MotorControlDevRef"=w22:T24)  [unwired: 9 in, 1 out]
  n146 = Bundle By Name(cluster=T5 {"Rollers Closed?"=FALSE, "Roller Mode"=enum."Manual", "Auto Roller State"=enum."Grab Tote", "Tote Inside?"=FALSE, "Intake State"=enum."Acquire Tote", "Left Ping Dist"=0.0, "Right Ping Dist"=0.0, "Potentiometer Cluster"={"Left Pot Zero"=0.0, "Right Pot Zero"=0.0, "Left Potentiometer"=0.0, "Right Potentiometer"=0.0, "Left Pot Non Zero"=0.0, "Right Pot Non Zero"=0.0}, "PING Decision"=enum."Acquire Tote", "Zero Complete?"=FALSE, "Left Arm Closed?"=FALSE, "Portrait?"=FALSE, "Right Arm Closed?"=FALSE, "Left Out"=0.0, "Right Out"=0.0, "Left Current"=0.0, "Right Current"=0.0, "Tote Load Complete?"=FALSE, "Untip Complete?"=FALSE, "Untip State"=enum."Idle", "Roller Safety Open"=FALSE} ("Roller State Indicators"), "Left Out"=w31, "Right Out"=w30, "Zero Complete?"=w37, "Rollers Closed?"=w38, "Auto Roller State"=w40, "Roller Mode"=w41, "Intake State"=w42, "Left Ping Dist"=w18, "Right Ping Dist"=w17, "PING Decision"=w39, "Portrait?"=w36, "Left Arm Closed?"=w35, "Right Arm Closed?"=w34, "Tote Load Complete?"=w27, "Untip Complete?"=w26, "Tote Inside?"=w13, "Left Current"=w12, "Right Current"=w11, "Potentiometer Cluster"=w10, "Roller Safety Open"=w1) -> (w46:T5)
  n147 = call <vilib>:"WPI_MotorControlRefNum Registry Get.vi"("refnum name"="Right Roller Motor") -> ("MotorControlDevRef"=w20:T24)  [unwired: 9 in, 1 out]
  n148 = disable-structure shown="Enabled" {
    disable-tunnel: w22 -> [w404 w406]
    disable-tunnel: w31 -> [w405 w409]
    disable-tunnel: w20 -> [w402 w407]
    disable-tunnel: w30 -> [w403 w408]
    frame Disabled {
      n149 = call <vilib>:"WPI_MotorControlSetOutput.vi"("Output"=w405, "MotorControlDevRef"=w404) -> ()  [unwired: 7 in, 3 out]
      n150 = call <vilib>:"WPI_MotorControlSetOutput.vi"("Output"=w403, "MotorControlDevRef"=w402) -> ()  [unwired: 7 in, 3 out]
    }
    frame Enabled {
      n151 = call "624FastTalonSetOutput.vi"("Output"=w409, "MotorControlDevRef"=w406) -> ()  [unwired: 8 in, 2 out]
      n152 = call "624FastTalonSetOutput.vi"("Output"=w408, "MotorControlDevRef"=w407) -> ()  [unwired: 8 in, 2 out]
    }
  }
  n153 = global write "Robot Global Data.vi" "Roller State Indicators"(w46) -> ()
  n154 = call <vilib>:"WPI_SolenoidRefNum Registry Get.vi"("refnum name"="Roller Piston") -> ("SolenoidDevRef"=w44:T22)  [unwired: 9 in, 1 out]
  n155 = call-poly <vilib>:"WPI_SolenoidSet.vi"("Value"=w38, "SolenoidDevRef"=w44) -> ()  [unwired: 8 in, 2 out]
